vi "Main.vi"() -> ()   [LabVIEW 2014, in "CML UI.lvlib"]
doc: "This template is based off of the Queued Message Handler design pattern and the Queued Message Handler project template that ships with LabVIEW.\n\nThe main difference is that the queue is private to this module and communication between modules is performed via Broadcast and Request events.\n\nRequest events are wrapped in public API methods and are handled in the Event Handling Loop (EHL) of this VI. Any module can register for Broadcast events sent by this module. The EHL generates messages based on user interface actions.\n\nThe Message Handling Loop (MHL) processes messages generated by the EHL, or by other messages. The messages are string values, so new messages can be added easily to the Message Cases case structure in the MHL. Each message cluster can also provide an optional value for Message Data, which is a variant that can be converted to whatever message-specific data is required.\n_____\nBased on Delacor QMH Project Template 4.0.0.47.\n_____\nBased on Delacor QMH Project Template 4.1.0.59."
uses:
  CML UI.lvlib
  <vilib>/Delacor/Delacor QMH/Libraries/Module Admin_class/Delacor_lib_QMH_Module Admin.lvclass
  Module Data--cluster.ctl
  Stop Argument--cluster.ctl
  <vilib>/Delacor/Delacor QMH/Libraries/Module Admin_class/Delacor_lib_QMH_Module Admin.lvclass/Delacor_lib_QMH_Module Admin.ctl
  <vilib>/Delacor/Delacor QMH/Libraries/Module Admin_class/Delacor_lib_QMH_Get External Launch.vi
  <vilib>/Delacor/Delacor QMH/Libraries/Message Queue_class/Delacor_lib_QMH_Enqueue Message (Single).vi
  <vilib>/Utility/error.llb/Error Cluster From Error Code.vi
  <vilib>/ErrorRing/Error Ring.xnode
  <vilib>/Delacor/Delacor QMH/Libraries/Message Queue_class/Delacor_lib_QMH_Message Queue.lvclass
  Settings Editor/Settings Editor.lvlib
  Acquisition/Acquisition.lvlib
  Logger/Logger.lvlib
panel:
  out "Logger Running?":bool
  out "Settings Editor Running?":bool
  out "Acquisition Running?":bool
  out "Data":waveform(dbl)[](graph)
  out "Calibrated?":bool
  in  "Calibrate":bool
  in  "Settings":bool
  in  "Start":bool
  in  "Stop":bool
  in  "Module Admin":refnum<class "Delacor_lib_QMH_Module Admin.lvclass">
  out "error out":errorcluster
  out "Status":string
  out "version":string
  # "Continuous Measurement Data Logger"
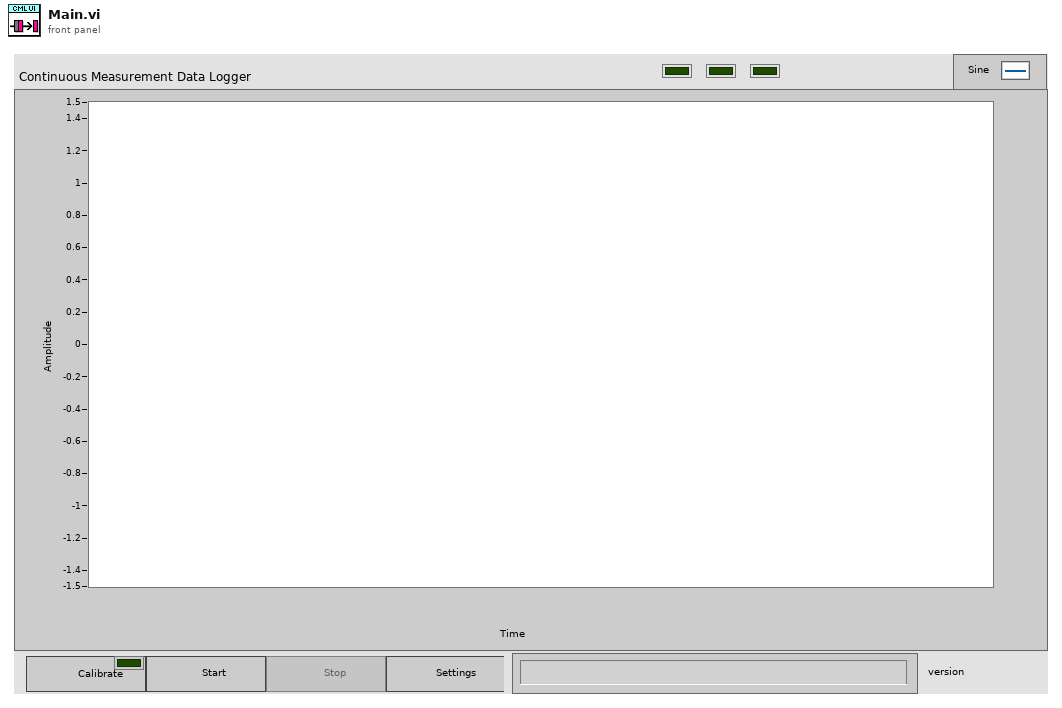
[diagram p1: front panel]
types:
  T1 = typedef "CML UI.lvlib/Request Events--cluster.ctl" = cluster{"Stop Module":refnum<user-event>, "Show Panel":refnum<user-event>, "Hide Panel":refnum<user-event>, "Get Module Execution Status":refnum<user-event>, "Show Diagram":refnum<user-event>}
  T2 = typedef "Settings Editor.lvlib/Broadcast Events--cluster.ctl" = cluster{"Module Did Init":refnum<user-event>, "Status Updated":refnum<user-event>, "Error Reported":refnum<user-event>, "Module Did Stop":refnum<user-event>, "Update Module Execution Status":refnum<user-event>, "Application Settings Updated":refnum<user-event>}
  T3 = typedef "Acquisition.lvlib/Broadcast Events--cluster.ctl" = cluster{"Module Did Init":refnum<user-event>, "Status Updated":refnum<user-event>, "Error Reported":refnum<user-event>, "Module Did Stop":refnum<user-event>, "Update Module Execution Status":refnum<user-event>, "Acquisition Started":refnum<user-event>, "Acquisition Stopped":refnum<user-event>, "Data Updated":refnum<user-event>, "Device Calibrated":refnum<user-event>}
  T4 = typedef "Logger.lvlib/Broadcast Events--cluster.ctl" = cluster{"Module Did Init":refnum<user-event>, "Status Updated":refnum<user-event>, "Error Reported":refnum<user-event>, "Module Did Stop":refnum<user-event>, "Update Module Execution Status":refnum<user-event>, "Logging Stopped":refnum<user-event>, "File Initialized":refnum<user-event>}
  T5 = typedef "CML UI.lvlib/Module Data--cluster.ctl" = cluster{"Status":string, "Measurement UI Controls":cluster{"Start Ref":refnum<vi>, "Stop Ref":refnum<vi>, "Settings Ref":refnum<vi>, "Status Ref":refnum<vi>, "Data Ref":refnum<vi>}}
  T6 = enum32{"invalid lock state", "Not Locked", "Locked (No Password)", "Password-protected"}
  T7 = typedef "CML UI.lvlib/Stop Argument--cluster.ctl" = cluster{"Origin":string, "Exit via Stop Module Req?":bool, "Wait for Module to stop?":bool}
  T8 = enum32{"Invalid", "Standard", "Closed", "Hidden", "Minimized", "Maximized"}
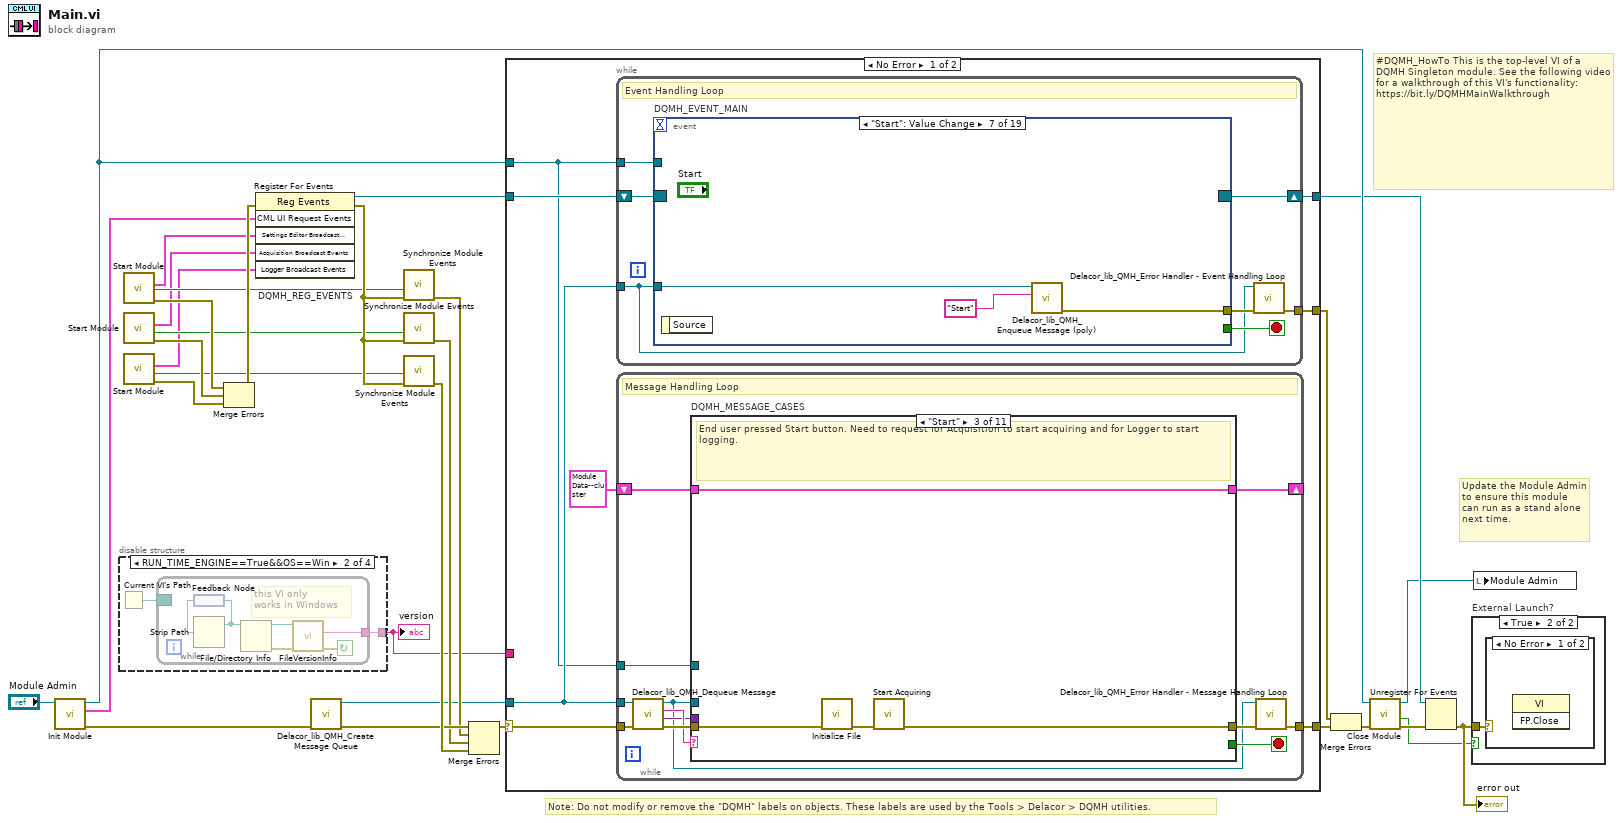
[diagram p0: block diagram]
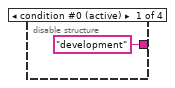
[diagram p2: hidden frame]
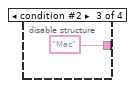
[diagram p3: hidden frame]
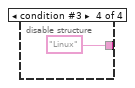
[diagram p4: hidden frame]
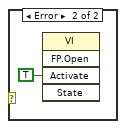
[diagram p6: hidden frame]
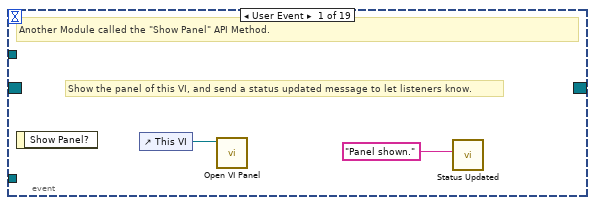
[diagram p7: hidden frame]
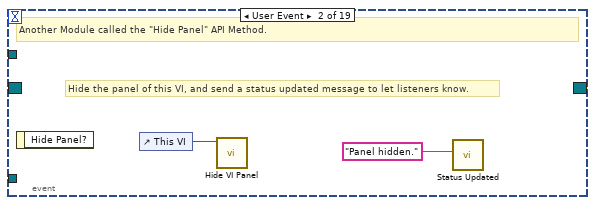
[diagram p8: hidden frame]
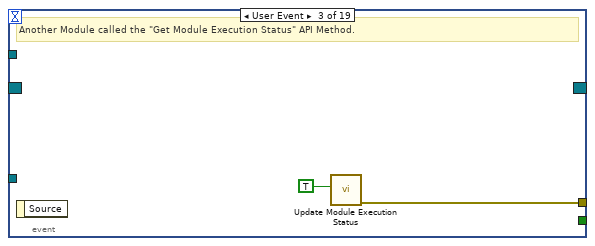
[diagram p9: hidden frame]
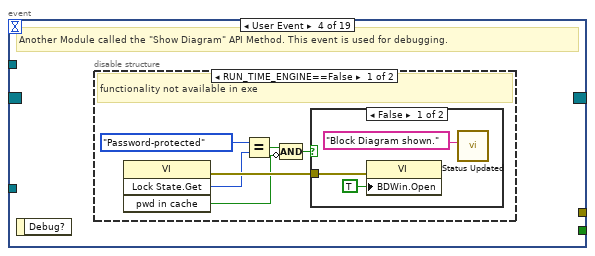
[diagram p10: hidden frame]
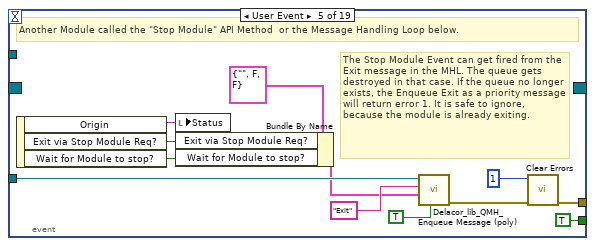
[diagram p13: hidden frame]
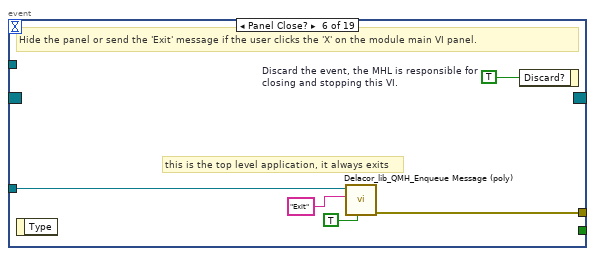
[diagram p14: hidden frame]
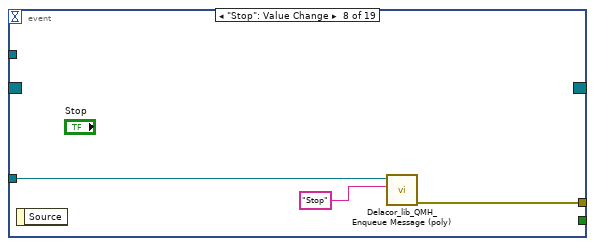
[diagram p15: hidden frame]
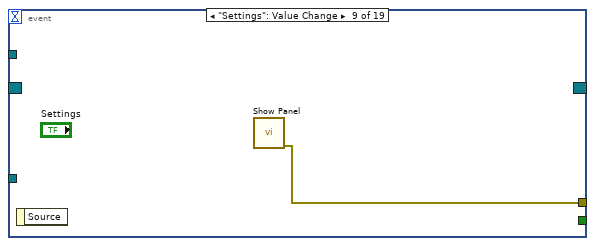
[diagram p16: hidden frame]
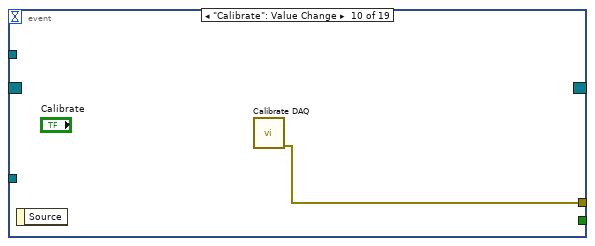
[diagram p17: hidden frame]
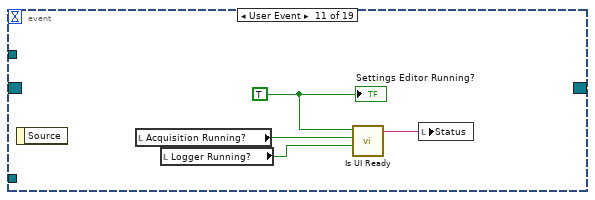
[diagram p18: hidden frame]
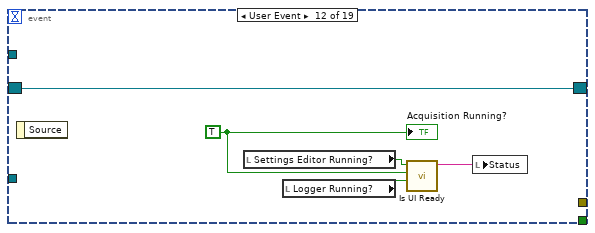
[diagram p19: hidden frame]
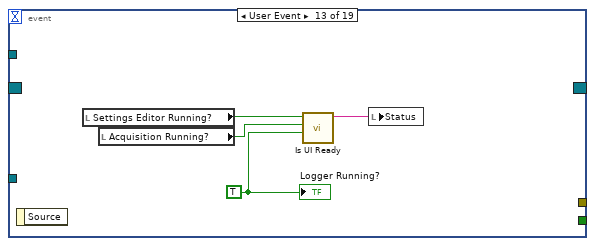
[diagram p20: hidden frame]
diagram:
  # "#DQMH_HowTo This is the top-level VI of a DQMH Singleton module. See the following video for a walkthrough of this VI's functionality: https://bit.ly/DQMHMainWalkthrough"
  # "Note: Do not modify or remove the \"DQMH\" labels on objects. These labels are used by the Tools > Delacor > DQMH utilities."
  # "Update the Module Admin to ensure this module can run as a stand alone next time."
  n1 = call "Init Module.vi"("Singleton Module Admin in"="Module Admin") -> ("error out"=w29:errorcluster, "CML UI Request Events"=w12:T1, "Singleton Module Admin out"=w15:refnum<class "Delacor_lib_QMH_Module Admin.lvclass">)  [unwired: 8 in]
  n2 = disable-structure "Conditional Disable Structure" shown="RUN_TIME_ENGINE==True&&OS==Win" {
    disable-tunnel: ["development" w33 "Mac" "Linux"] -> w1
    frame condition #0 (active) {
    }
    frame condition #1 {
      n3 = Current VI's Path() -> (path=w34:path)
      n4 = while {
        border: w34 -> [_]
        tunnel: [w35] -> w33
        stop <- w39 continue-if-true
        # "this VI only \nworks in Windows"
        n5 = feedback #1() -> (w38:path)
        n6 = Strip Path(path=w38) -> (stripped path=w37:path)  [unwired: 1 out]
        n7 = feedback-in #1(w37) -> ()
        n8 = File/Directory Info(path=w37) -> (path out=w36:path, error out=w40:errorcluster)  [unwired: 1 in, 5 out]
        n9 = call <vilib>:"FileVersionInfo.vi"("error in (no error)"=w40, "Application Path in"=w36) -> ("error out"=w39:errorcluster, "File Version Info"=w35:string)  [unwired: 6 in, 2 out]
      }
    }
    frame condition #2 {
    }
    frame condition #3 {
    }
  }
  "version" <- w1
  n10 = call "Start Module.vi"() -> ("error out"=w20:errorcluster, "Wait for Event Sync?"=w7:bool, "Settings Editor Broadcast Events"=w6:T2)  [unwired: 8 in, 1 out]
  n11 = call "Start Module.vi"() -> ("error out"=w19:errorcluster, "Wait for Event Sync?"=w4:bool, "Acquisition Broadcast Events"=w5:T3)  [unwired: 8 in, 1 out]
  n12 = call "Start Module.vi"() -> ("error out"=w18:errorcluster, "Wait for Event Sync?"=w2:bool, "Logger Broadcast Events"=w3:T4)  [unwired: 8 in, 1 out]
  n13 = Merge Errors(w20, w19, w18) -> (w17:errorcluster)
  n14 = register-events "DQMH_REG_EVENTS"(error in=w17, w12, w6, w5, w3) -> (reference out=w13:refnum<event-registration>, error out=w16:errorcluster)  [unwired: 1 in]
  n15 = call <vilib>:"Delacor_lib_QMH_Create Message Queue.vi"("error in (no error)"=w29) -> ("error out"=w24:errorcluster, "Message Queue"=w11:refnum<class "Delacor_lib_QMH_Message Queue.lvclass">)  [unwired: 9 in]
  n16 = call "Synchronize Module Events.vi"("error in (no error)"=w16, "Wait for Event Sync?"=w7) -> ("error out"=w22:errorcluster)  [unwired: 9 in]
  n17 = call "Synchronize Module Events.vi"("error in (no error)"=w16, "Wait for Event Sync?"=w4) -> ("error out"=w21:errorcluster)  [unwired: 9 in]
  n18 = call "Synchronize Module Events.vi"("error in (no error)"=w16, "Wait for Event Sync?"=w2) -> ("error out"=w31:errorcluster)  [unwired: 9 in]
  n19 = Merge Errors(w24, w22, w21, w31) -> (w23:errorcluster)
  n20 = case shown="No Error" w23 {
    selector: w23 -> [w48 w262]
    tunnel: [w50 w262] -> w30
    tunnel: [w47 w259] -> w14
    tunnel: w13 -> [w45 w259]
    tunnel: w11 -> [w44 w252]
    tunnel: [w49 _] -> w27
    tunnel: w15 -> [w43 w255]
    tunnel: w1 -> [_ _]
    frame No Error {
      n21 = while {
        tunnel: w44 -> [w51]
        shift-right: [w54] -> w47
        shift-left: w45 -> [w55]
        tunnel: [w56] -> w49
        tunnel: w43 -> [w52]
        stop <- w53 stop-if-true
        # "Event Handling Loop"
        n22 = event "DQMH_EVENT_MAIN" shown="[6] \"Start\": Value Change" {
          selector: w55 -> [_ _ _ _ _ _ _ _ _ _ _ w106 _ _ _ _ _ _ _]
          dyn-events: [_ _ _ _ _ _ _ _ _ _ _ w106 _ _ _ _ _ _ _] -> w54
          timeout: _ -> [_ _ _ _ _ _ _ _ _ _ _ _ _ _ _ _ _ _ _]
          tunnel: [_ _ _ _ TRUE ("Discard?") _ _ _ _ _ _ _ _ _ _ _ _ _ _] -> w53
          tunnel: w51 -> [_ _ _ _ w80 w87 w90 w93 _ _ _ _ _ _ _ w118 w120 _ _]
          tunnel: [_ _ w63 _ w83 w89 w92 w95 w96 w97 _ _ _ _ w116 _ _ _ _] -> w57
          tunnel: w52 -> [_ _ _ _ _ _ _ _ _ _ _ _ _ _ _ _ _ _ _]
          event User Event {
            # "Show the panel of this VI, and send a status updated message to let listeners know."
            # "Another Module called the \"Show Panel\" API Method."
            n23 = event-data() -> ()  [unwired: 1 in, 1 out]
            n24 = control-ref of="This VI"() -> (w59:refnum<vi>)
            n25 = call "Open VI Panel.vi"("VI"=w59) -> ()  [unwired: 10 in, 1 out]
            n26 = call "Status Updated.vi"("Status"="Panel shown." ("format string")) -> ()  [unwired: 10 in, 1 out]
          }
          event User Event {
            # "Hide the panel of this VI, and send a status updated message to let listeners know."
            # "Another Module called the \"Hide Panel\" API Method."
            n27 = event-data() -> ()  [unwired: 1 in, 1 out]
            n28 = control-ref of="This VI"() -> (w61:refnum<vi>)
            n29 = call "Hide VI Panel.vi"("VI"=w61) -> ()  [unwired: 10 in, 1 out]
            n30 = call "Status Updated.vi"("Status"="Panel hidden." ("format string")) -> ()  [unwired: 10 in, 1 out]
          }
          event User Event {
            # "Another Module called the \"Get Module Execution Status\" API Method."
            n31 = event-data() -> ()  [unwired: 1 in, 1 out]
            n32 = call "Update Module Execution Status.vi"("Running?"=TRUE) -> ("error out"=w63:errorcluster)  [unwired: 10 in]
          }
          event User Event {
            # "Another Module called the \"Show Diagram\" API Method. This event is used for debugging."
            n33 = event-data() -> ()  [unwired: 1 in, 1 out]
            n34 = disable-structure shown="RUN_TIME_ENGINE==False" {
              frame condition #0 (active) {
                # "functionality not available in exe"
                n35 = invoke on="Invoke Node" class="VI" method="Lock State.Get"() -> (error out=w69:errorcluster, "Get Lock State"=w68:T6, "pwd in cache"=w65:bool)  [unwired: 4 in, 1 out]
                n36 = Equal?(x=T6."Password-protected", y=w68) -> (x = y?=w66:bool)
                n37 = Compound Arithmetic op=AND(w66, invert w65) -> (w64:bool)
                n38 = case shown="False" w64 {
                  tunnel: w69 -> [w72 _]
                  frame False {
                    n39 = property on="Property Node" class="VI"(error in=w72, "BDWin.Open"=TRUE ("Block Diagram Window:Open")) -> ()  [unwired: 1 in, 2 out]
                    n40 = call "Status Updated.vi"("Status"="Block Diagram shown." ("format string")) -> ()  [unwired: 10 in, 1 out]
                  }
                  frame True {
                    # "Password-protected VI, and the password is not in the cache. Do not show the diagram."
                  }
                }
              }
              frame condition #1 {
              }
            }
          }
          event User Event {
            # "The Stop Module Event can get fired from the Exit message in the MHL. The queue gets destroyed in that case. If the queue no longer exists, the Enqueue Exit as a priority message will return error 1. It is safe to ignore, because the module is already exiting."
            # "Another Module called the \"Stop Module\" API Method  or the Message Handling Loop below."
            n41 = event-data() -> ("Origin"=w79:string, "Exit via Stop Module Req?"=w75:bool, "Wait for Module to stop?"=w74:bool)  [unwired: 1 in]
            n42 = local write "Status"(w79) -> ()
            n43 = Bundle By Name(cluster=T7 {"Origin"="", "Exit via Stop Module Req?"=FALSE, "Wait for Module to stop?"=FALSE} ("Stop Argument"), "Exit via Stop Module Req?"=w75, "Wait for Module to stop?"=w74) -> (w73:T7)
            n44 = call-poly <vilib>:"Delacor_lib_QMH_Enqueue Message (poly).vi"("Priority Message? (F)"=TRUE, "Message Data"=w73, "Message"="Exit", "Message Queue in"=w80) -> ("error out"=w84:errorcluster)  [unwired: 6 in, 1 out]
            n45 = call <vilib>:"Clear Errors.vi"("error in (no error)"=w84, "specific error code to clear (0: all)"=1) -> ("error out"=w83:errorcluster)  [unwired: 4 in, 1 out]
          }
          event Panel Close? {
            w88 = TRUE  # Discard the event, the MHL is responsible for closing and stopping this VI.
            # "this is the top level application, it always exits"
            # "Hide the panel or send the 'Exit' message if the user clicks the 'X' on the module main VI panel."
            n46 = event-data() -> ()  [unwired: 1 in, 1 out]
            n47 = call-poly <vilib>:"Delacor_lib_QMH_Enqueue Message (poly).vi"("Priority Message? (F)"=TRUE, "Message"="Exit", "Message Queue in"=w87) -> ("error out"=w89:errorcluster)  [unwired: 7 in, 1 out]
            n48 = event-data ("Event Filter Node")("Discard?"=w88) -> ()  [unwired: 1 in, 1 out]
          }
          event "Start": Value Change {
            n49 = event-data() -> ()  [unwired: 1 in, 1 out]
            n50 = call-poly <vilib>:"Delacor_lib_QMH_Enqueue Message (poly).vi"("Message"="Start", "Message Queue in"=w90) -> ("error out"=w92:errorcluster)  [unwired: 8 in, 1 out]
          }
          event "Stop": Value Change {
            n51 = event-data() -> ()  [unwired: 1 in, 1 out]
            n52 = call-poly <vilib>:"Delacor_lib_QMH_Enqueue Message (poly).vi"("Message"="Stop", "Message Queue in"=w93) -> ("error out"=w95:errorcluster)  [unwired: 8 in, 1 out]
          }
          event "Settings": Value Change {
            n53 = event-data() -> ()  [unwired: 1 in, 1 out]
            n54 = call "Show Panel.vi"() -> ("error out"=w96:errorcluster)  [unwired: 11 in]
          }
          event "Calibrate": Value Change {
            n55 = event-data() -> ()  [unwired: 1 in, 1 out]
            n56 = call "Calibrate DAQ.vi"() -> ("error out"=w97:errorcluster)  [unwired: 11 in]
          }
          event User Event {
            w99 = TRUE ("Settings Editor Running?")
            n57 = event-data() -> ()  [unwired: 1 in, 1 out]
            n58 = local read "Acquisition Running?"() -> (w101:bool)
            n59 = local read "Logger Running?"() -> (w100:bool)
            n60 = call "Is UI Ready.vi"("Logger Running?"=w100, "Acquisition Running?"=w101, "Settings Editor Running?"=w99) -> ("Status"=w98:string)  [unwired: 8 in]
            n61 = local write "Status"(w98) -> ()
            "Settings Editor Running?" <- w99
          }
          event User Event {
            w104 = TRUE ("Acquisition Running?")
            n62 = event-data() -> ()  [unwired: 1 in, 1 out]
            n63 = local read "Settings Editor Running?"() -> (w103:bool)
            n64 = local read "Logger Running?"() -> (w102:bool)
            n65 = call "Is UI Ready.vi"("Logger Running?"=w102, "Acquisition Running?"=w104, "Settings Editor Running?"=w103) -> ("Status"=w105:string)  [unwired: 8 in]
            n66 = local write "Status"(w105) -> ()
            "Acquisition Running?" <- w104
          }
          event User Event {
            w109 = TRUE ("Logger Running?")
            n67 = event-data() -> ()  [unwired: 1 in, 1 out]
            n68 = local read "Settings Editor Running?"() -> (w108:bool)
            n69 = local read "Acquisition Running?"() -> (w107:bool)
            n70 = call "Is UI Ready.vi"("Logger Running?"=w109, "Acquisition Running?"=w107, "Settings Editor Running?"=w108) -> ("Status"=w110:string)  [unwired: 8 in]
            n71 = local write "Status"(w110) -> ()
            "Logger Running?" <- w109
          }
          event User Event {
            n72 = event-data() -> ("Status"=w111:string)  [unwired: 1 in]
            "Status" <- w111
            n73 = call "Status Updated.vi"("Status"=w111) -> ()  [unwired: 10 in, 1 out]
          }
          event User Event {
            n74 = event-data() -> ("Error"=w116:errorcluster, "Module Name"=w114:string)  [unwired: 1 in, 1 out]
            n75 = Unbundle By Name(w116) -> ("code"=w115:i32)
            n76 = Format Into String(format string="Error %d at %s", w115, w114) -> (resulting string=w113:string)  [unwired: 2 in, 1 out]
            n77 = local write "Status"(w113) -> ()
          }
          event User Event {
            n78 = event-data() -> ()  [unwired: 1 in, 1 out]
            n79 = call-poly <vilib>:"Delacor_lib_QMH_Enqueue Message (poly).vi"("Message"="Acquisition Started Interlocks", "Message Queue in"=w118) -> ()  [unwired: 8 in, 2 out]
          }
          event User Event {
            n80 = event-data() -> ()  [unwired: 1 in, 1 out]
            n81 = call-poly <vilib>:"Delacor_lib_QMH_Enqueue Message (poly).vi"("Message"="Acquisition Stopped Interlocks", "Message Queue in"=w120) -> ()  [unwired: 8 in, 2 out]
          }
          event User Event {
            n82 = event-data() -> ("Graph Data"=→"Data":waveform(dbl)[])  [unwired: 1 in]
          }
          event User Event {
            n83 = event-data() -> ()  [unwired: 1 in, 1 out]
            "Calibrated?" <- TRUE ("Calibrated?")
          }
        }
        n84 = call-dynamic "Delacor_lib_QMH_Error Handler - Event Handling Loop.vi"("error in (no error)"=w57, "Message Queue in"=w51) -> ("dup error in"=w56:errorcluster)  [unwired: 8 in, 1 out]
      }
      n85 = while {
        tunnel: w44 -> [w125]
        shift-right: [w129] -> _
        shift-left: T5 {"Status"="", "Measurement UI Controls"={"Start Ref"=refnum, "Stop Ref"=refnum, "Settings Ref"=refnum, "Status Ref"=refnum, "Data Ref"=refnum}} ("Data Cluster") -> [w130]
        tunnel: w48 -> [w133]
        tunnel: [w131] -> w50
        tunnel: w43 -> [w123]
        stop <- w128 stop-if-true
        # "Message Handling Loop"
        n86 = call-dynamic "Delacor_lib_QMH_Dequeue Message.vi"("error in (no error)"=w133, "Message Queue in"=w125) -> ("error out"=w132:errorcluster, "Message Data"=w126:variant, "Message"=w127:string, "Message Queue out"=w124:refnum<class "Delacor_lib_QMH_Message Queue.lvclass">)  [unwired: 6 in]
        n87 = case "DQMH_MESSAGE_CASES" shown="\"Start\"" w127 {
          selector: w127 -> [_ _ _ _ _ _ _ _ _ _ w239]
          tunnel: w124 -> [_ _ _ _ _ _ _ _ w203 w230 _]
          tunnel: w132 -> [w165 w169 w172 w182 w185 w195 w198 w200 w210 w235 w241]
          tunnel: [w163 w169 w171 w182 w184 w195 w197 w200 w206 w219 w242] -> w134
          tunnel: w130 -> [w154 w168 w170 w174 w183 w187 w196 w199 w205 w229 w240]
          tunnel: [w143 w168 w170 w174 w183 w187 w196 w199 w205 w229 w240] -> w129
          tunnel: [_ _ _ _ _ _ _ _ _ w228 _] -> w128
          tunnel: w126 -> [_ _ _ _ _ _ _ _ w204 w227 _]
          tunnel: w123 -> [w155 _ _ _ _ _ _ _ w202 w222 _]
          frame "Initialize" {
            w149 = "Initial Message" ("Initial Message")
            # "Enable: Start, Settings\nDisable: Stop"
            # "Initialize - Any operation that needs to be done before the module can receive messages. Synchronize Caller Events.vi will inform Start Module.vi that the module has launched and is ready to receive messages. Module Did Init.vi will broadcast that the module initialized."
            n88 = call "Synchronize Caller Events.vi"("error in (no error)"=w165, "Singleton Module Admin in"=w155) -> ("error out"=w164:errorcluster, "Singleton Module Admin out"=w151:refnum<class "Delacor_lib_QMH_Module Admin.lvclass">)  [unwired: 8 in]
            n89 = property on="Property Node" class="Module Admin"(reference=w151) -> ("Accessors:External Launch"=w159:bool)  [unwired: 1 in, 2 out]
            n90 = property on="Data" class="WFChart (strict)"("History Data"=waveform(dbl)[][] []) -> ()  [unwired: 2 in, 2 out]
            n91 = control-ref of="Data"() -> (w144:refnum<vi>)
            n92 = local write "Calibrated?"(FALSE ("Calibrated?")) -> ()
            n93 = control-ref of="Start"() -> (w148:refnum<vi>)
            n94 = control-ref of="Stop"() -> (w147:refnum<vi>)
            n95 = control-ref of="Settings"() -> (w146:refnum<vi>)
            n96 = control-ref of="Status"() -> (w145:refnum<vi>)
            n97 = Select(t=T8."Hidden" ("State"), s=w159, f=T8."Standard" ("State")) -> (s? t:f=w156:T8)
            n98 = call "Module Name--constant.vi"() -> ("Module Name"=w162:string)  [unwired: 11 in]
            n99 = Bundle By Name(cluster=w154, "Measurement UI Controls.Start Ref"=w148, "Measurement UI Controls.Stop Ref"=w147, "Measurement UI Controls.Settings Ref"=w146, "Measurement UI Controls.Status Ref"=w145, "Measurement UI Controls.Data Ref"=w144, "Status"=w149) -> (w143:T5)
            n100 = local write "Status"(w149) -> ()
            n101 = property on="Property Node" class="VI"("Front Panel.Title"=w162) -> (reference out=w161:refnum<vi>, error out=w167:errorcluster)  [unwired: 2 in]
            n102 = invoke on="Invoke Node" class="VI" method="FP.Open"(reference=w161, error in=w167, "State"=w156) -> (reference out=w160:refnum<vi>, error out=w166:errorcluster)  [unwired: 2 in, 3 out]
            n103 = Unbundle By Name(w143) -> ("Measurement UI Controls.Start Ref"=w142:refnum<vi>, "Measurement UI Controls.Settings Ref"=w141:refnum<vi>, "Measurement UI Controls.Stop Ref"=w138:refnum<vi>)
            n104 = call "Module Name--constant.vi"() -> ("Module Name"=w152:string)  [unwired: 11 in]
            n105 = invoke on="Invoke Node" class="VI" method="FP.Center"(reference=w160, error in=w166) -> ()  [unwired: 1 in, 3 out]
            n106 = Build Array(w142, w141) -> (w140:refnum<vi>[])
            n107 = Build Array(w138) -> (w137:refnum<vi>[])
            n108 = call "Module Did Init.vi"("error in (no error)"=w164, "Initialized?"=TRUE, "Origin"=w152) -> ("error out"=w163:errorcluster)  [unwired: 8 in]
            n109 = call "Set Enable State on Multiple Controls.vi"("Enable?"=FALSE, "Controls"=w137) -> ()  [unwired: 10 in]
            n110 = call "Set Enable State on Multiple Controls.vi"("Enable?"=TRUE, "Controls"=w140) -> ()  [unwired: 10 in]
          }
          frame "--- Module Specific ---" {
            # "Separator -- The following cases handle messages specific to this Module."
          }
          frame "Start" {
            # "End user pressed Start button. Need to request for Acquisition to start acquiring and for Logger to start logging."
            n111 = call "Initialize File.vi"("error in (no error)"=w172) -> ("error out"=w173:errorcluster)  [unwired: 8 in, 2 out]
            n112 = call "Start Acquiring.vi"("error in (no error)"=w173) -> ("error out"=w171:errorcluster)  [unwired: 8 in, 2 out]
          }
          frame "Acquisition Started Interlocks" {
            # "Enable: Stop\nDisable: Start, Settings"
            n113 = Unbundle By Name(w174) -> ("Measurement UI Controls.Stop Ref"=w181:refnum<vi>, "Measurement UI Controls.Start Ref"=w176:refnum<vi>, "Measurement UI Controls.Settings Ref"=w175:refnum<vi>)
            n114 = Build Array(w181) -> (w180:refnum<vi>[])
            n115 = Build Array(w176, w175) -> (w177:refnum<vi>[])
            n116 = call "Set Enable State on Multiple Controls.vi"("Enable?"=TRUE, "Controls"=w180) -> ()  [unwired: 10 in]
            n117 = call "Set Enable State on Multiple Controls.vi"("Enable?"=FALSE, "Controls"=w177) -> ()  [unwired: 10 in]
          }
          frame "Stop" {
            # "End user pressed Stop button. Need to request for Acquisition to stop acquiring and for Logger to stop logging."
            n118 = call "Stop Acquiring.vi"("error in (no error)"=w185) -> ("error out"=w186:errorcluster)  [unwired: 10 in]
            n119 = call "Stop Logging.vi"("error in (no error)"=w186) -> ("error out"=w184:errorcluster)  [unwired: 10 in]
          }
          frame "Acquisition Stopped Interlocks" {
            # "Enable: Start, Settings\nDisable: Stop"
            n120 = Unbundle By Name(w187) -> ("Measurement UI Controls.Stop Ref"=w192:refnum<vi>, "Measurement UI Controls.Start Ref"=w191:refnum<vi>, "Measurement UI Controls.Settings Ref"=w190:refnum<vi>)
            n121 = Build Array(w192) -> (w194:refnum<vi>[])
            n122 = Build Array(w191, w190) -> (w189:refnum<vi>[])
            n123 = call "Set Enable State on Multiple Controls.vi"("Enable?"=FALSE, "Controls"=w194) -> ()  [unwired: 10 in]
            n124 = call "Set Enable State on Multiple Controls.vi"("Enable?"=TRUE, "Controls"=w189) -> ()  [unwired: 10 in]
          }
          frame "---Copy This Frame---" {
            # "Duplicate this frame when creating new messages.  Change this comment in the duplicated frame to describe this message."
            n125 = Merge Errors(w198) -> (w197:errorcluster)
          }
          frame "--- Exit and Error Handling---" {
            # "Separator - The following cases handle errors and exit messages."
          }
          frame "Error" {
            # "Error - Check the error message data and respond accordingly. This message is sent by the \"Error Handler\" VIs at the end of each loop in this application."
            n126 = property on="Property Node" class="Module Admin"(reference=w202) -> ("Accessors:External Launch"=w201:bool)  [unwired: 1 in, 2 out]
            n127 = Variant To Data(error in=w210, type=errorcluster {"status"=FALSE, "code"=0, "source"=""} ("error constant"), Variant=w204) -> (data=w211:errorcluster, error out=w208:errorcluster)
            n128 = call "Error Reported.vi"("Error"=w211) -> ()  [unwired: 10 in, 1 out]
            n129 = case shown="False" w201 {
              tunnel: [w216 _] -> w207
              tunnel: w203 -> [w214 _]
              tunnel: w211 -> [w215 _]
              frame False {
                # "If the module is running standalone, then pop up an error dialog and call the \"Exit\" message."
                n130 = call <vilib>:"Simple Error Handler.vi"("error in (no error)"=w215) -> ()  [unwired: 4 in, 5 out]
                n131 = call-poly <vilib>:"Delacor_lib_QMH_Enqueue Message (poly).vi"("Priority Message? (F)"=TRUE, "Message"="Exit", "Message Queue in"=w214) -> ("error out"=w216:errorcluster)  [unwired: 7 in, 1 out]
              }
              frame True {
                # "If the module was launched externally, calling the Error Reported broadcast VI is the only action performed by the \"Error\" message. The module's caller can then process the error appropriately."
              }
            }
            n132 = Merge Errors(w208, w207) -> (w206:errorcluster)
            n133 = local write "error out"(w206) -> ()
          }
          frame "Exit" {
            w221 = TRUE ("Wait for Module to Stop? (F)")
            w226 = 91  # 91: not all Exit messages will have an argument
            w228 = TRUE  # Stop the VI
            # "DAQ and LOG modules use the settings editor. CML UI module waits for both modules to completely stop before stopping the settings editor."
            # "Release the message queue reference"
            # "Exit - Exit the application."
            n134 = Variant To Data(error in=w235, type=T7 {"Origin"="", "Exit via Stop Module Req?"=FALSE, "Wait for Module to stop?"=FALSE} ("Stop Argument"), Variant=w227) -> (data=w224:T7, error out=w232:errorcluster)
            n135 = call <vilib>:"Clear Errors.vi"("error in (no error)"=w232, "specific error code to clear (0: all)"=w226) -> ("error out"=w234:errorcluster)  [unwired: 4 in, 1 out]
            n136 = control-ref of="This VI"() -> (w223:refnum<vi>)
            n137 = call "Module Name--constant.vi"() -> ("Module Name"=w220:string)  [unwired: 11 in]
            n138 = call "Handle Exit.vi"("Stop Argument"=w224, "Admin in"=w222, "VI reference"=w223) -> ("error out"=w231:errorcluster)  [unwired: 7 in, 1 out]
            n139 = call "Stop Module.vi"("Wait for Module to Stop? (F)"=w221, "Origin"=w220) -> ("error out"=w218:errorcluster)  [unwired: 9 in]
            n140 = call "Stop Module.vi"("Wait for Module to Stop? (F)"=w221, "Origin"=w220) -> ("error out"=w217:errorcluster)  [unwired: 9 in]
            n141 = call-dynamic "Delacor_lib_QMH_Release Message Queue.vi"("error in (no error)"=w234, "Message Queue"=w230) -> ("error out"=w233:errorcluster)  [unwired: 9 in]
            n142 = Merge Errors(w218, w217) -> (w236:errorcluster)
            n143 = Merge Errors(w233, w231) -> (w219:errorcluster)
            n144 = call <vilib>:"Clear Errors.vi"("error in (no error)"=w236) -> ("error out"=w237:errorcluster)  [unwired: 5 in, 1 out]
            n145 = call "Stop Module.vi"("error in (no error)"=w237, "Wait for Module to Stop? (F)"=w221, "Origin"=w220) -> ()  [unwired: 8 in, 1 out]
          }
          frame Default {
            # "'Default' case only runs if there is a message that isn't defined in any of the other cases.  Output a programming error."
            n146 = call "Module Name--constant.vi"() -> ("Module Name"=w238:string)  [unwired: 11 in]
            n147 = xnode ("Error Ring")("parameter 0"=w239, "parameter 1"=w238) -> ("error out"=w243:errorcluster)
            n148 = Merge Errors(w241, w243) -> (w242:errorcluster)
          }
        }
        n149 = call-dynamic "Delacor_lib_QMH_Error Handler - Message Handling Loop.vi"("error in (no error)"=w134, "Message Queue in"=w124) -> ("dup error in"=w131:errorcluster)  [unwired: 8 in, 1 out]
      }
    }
    frame Error {
      w254 = TRUE ("Wait for Module to Stop? (F)")
      # "Synchronize Caller Events.vi will inform Start Module.vi that the module has launched and will let the code calling Start Module.vi register for broadcasts and would permit the caller receive the broadcast that an error occurred at launch time."
      n150 = call "Synchronize Caller Events.vi"("Singleton Module Admin in"=w255) -> ("error out"=w260:errorcluster)  [unwired: 9 in, 1 out]
      n151 = call "Module Name--constant.vi"() -> ("Module Name"=w258:string)  [unwired: 11 in]
      n152 = call "Module Name--constant.vi"() -> ("Module Name"=w253:string)  [unwired: 11 in]
      n153 = call-dynamic "Delacor_lib_QMH_Release Message Queue.vi"("Message Queue"=w252) -> ()  [unwired: 10 in, 1 out]
      n154 = call "Stop Module.vi"("Wait for Module to Stop? (F)"=w254, "Origin"=w253) -> ()  [unwired: 9 in, 1 out]
      n155 = call "Stop Module.vi"("Wait for Module to Stop? (F)"=w254, "Origin"=w253) -> ()  [unwired: 9 in, 1 out]
      n156 = call "Stop Module.vi"("Wait for Module to Stop? (F)"=w254, "Origin"=w253) -> ()  [unwired: 9 in, 1 out]
      n157 = Format Into String(format string="An error occurred during initialization. %s is no longer running.", w258) -> (resulting string=w256:string)  [unwired: 2 in, 1 out]
      n158 = Merge Errors(w262, w260) -> (w261:errorcluster)
      n159 = call "Error Reported.vi"("Additional Information"=w256, "Error"=w261) -> ()  [unwired: 9 in, 1 out]
    }
  }
  n160 = Merge Errors(w27, w30) -> (w26:errorcluster)
  n161 = call "Close Module.vi"("error in (no error)"=w26, "Module Admin in"=w15) -> ("error out"=w28:errorcluster, "External Launch"=w8:bool, "Module Admin out"=w9:refnum<class "Delacor_lib_QMH_Module Admin.lvclass">)  [unwired: 7 in]
  n162 = Unregister For Events(event registration refnum=w14, error in=w28) -> (error out=w25:errorcluster)
  "error out" <- w25
  n163 = case "External Launch?" shown="True" w8 {
    tunnel: w25 -> [_ w263]
    frame False {
    }
    frame True {
      n164 = case shown="No Error" w263 {
        frame No Error {
          n165 = invoke class="VI" method="FP.Close"() -> ()  [unwired: 3 in, 3 out]
        }
        frame Error {
          n166 = invoke on="Invoke Node" class="VI" method="FP.Open"("Activate"=TRUE ("Activate?")) -> ()  [unwired: 4 in, 5 out]
        }
      }
    }
  }
  n167 = local write "Module Admin"(w9) -> ()
